vi "QMH_Send_notifier.vi"(8 "error in (no error)":errorcluster, 10 "Payload":variant, 11 "Message":T1) -> (0 "error out":errorcluster)   [LabVIEW 2021, in "Framework_lib.lvlib"]
uses:
  Framework_lib.lvlib
  QMH_producer_enum.ctl
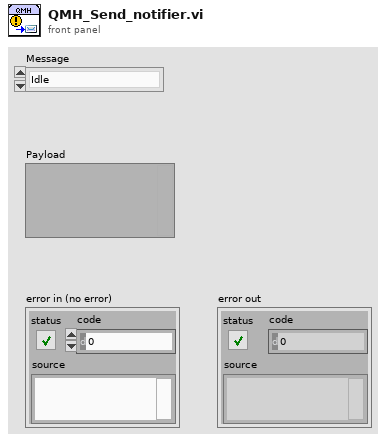
[diagram p1: front panel]
types:
  T1 = typedef "Framework_lib.lvlib/QMH_producer_enum.ctl" = enum16{"Idle", "Initialize", "Shutdown", "ERROR", "Stop"}
  T2 = typedef "Framework_lib.lvlib/QMH_references.ctl" = cluster{"Consumer_SUT":refnum<queue>, "Consumer_annotation":refnum<queue>, "compute_results":refnum<queue>, "Notifier":refnum<notifier>}
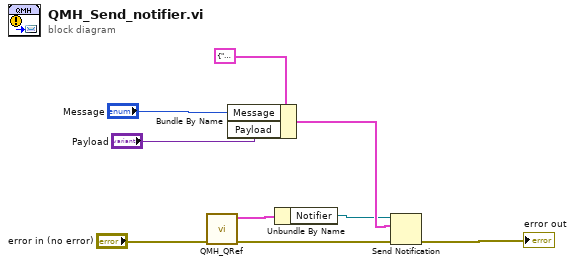
[diagram p0: block diagram]
diagram:
  n1 = call "QMH_QRef.vi"("error in (no error)"="error in (no error)") -> ("error out"=w3:errorcluster, "Cluster Out"=w2:T2)  [unwired: 8 in, 1 out]
  n2 = Bundle By Name(cluster=cluster{"Message":T1, "Payload":variant} {"Message"=enum."Shutdown", "Payload"=variant} ("notification"), "Message"="Message", "Payload"="Payload") -> (w6:cluster{"Message":T1, "Payload":variant})
  n3 = Unbundle By Name(w2) -> ("Notifier"=w1:refnum<notifier>)
  n4 = Send Notification(notification=w6, notifier=w1, error in (no error)=w3) -> (error out=→"error out":errorcluster)  [unwired: 1 out]
